vi "Convert C to F.vi"(1 "Degrees Celsius":dbl) -> (0 "Degrees Fahrenheit":dbl)   [LabVIEW 2014]
doc: "This VI converts a Celsius reading to a Fahrenheit reading."
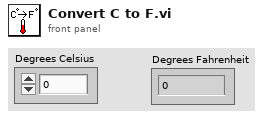
[diagram p1: front panel]
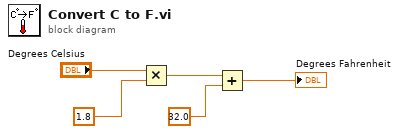
[diagram p0: block diagram]
diagram:
  n1 = Multiply(x="Degrees Celsius", y=1.8) -> (x*y=w3:dbl)
  n2 = Add(x=w3, y=32.0) -> (x+y=→"Degrees Fahrenheit":dbl)
